vi "SortAndNormalise.vi"(0 "Resampler":T1, 1 "ResampleToN":i32=12, 2 "ResampleHeights":dbl[](array[numeric])=[25.4, 38.1, 50.8, 76.2, 101.6, 127.0, 152.4, 203.2, 254.0, 304.8, 406.4, 508.0, 609.6, 812.8, 1219.2, 1524.0], 5 "Plot Array In":cluster{"Array":dbl[], "Array":dbl[]}[](array[cluster]), 7 "LegendsIn":string[](array[string]), 9 "Use for:":T2(array[ring])=[enum."\nU", enum."\nLambda", enum."\nTI", enum."\nSigma"], 12 "Zref":dbl) -> (4 "SortedLegends":string[](array[string]), 6 "SortedData":cluster{"Array":dbl[], "Array":dbl[]}[](array[cluster]), 8 "LeftGraph":cluster{"Array":dbl[], "Array":dbl[]}[](array[cluster]), 10 "RightGraph":cluster{"Array":dbl[], "Array":dbl[]}[](array[cluster]), 14 "UzClusterOutput":cluster{"Array":dbl[], "Array":dbl[]})   [LabVIEW 2021]
uses:
  Resampler.ctl
panel:
  # "Fit using values at  measurement Z heights"
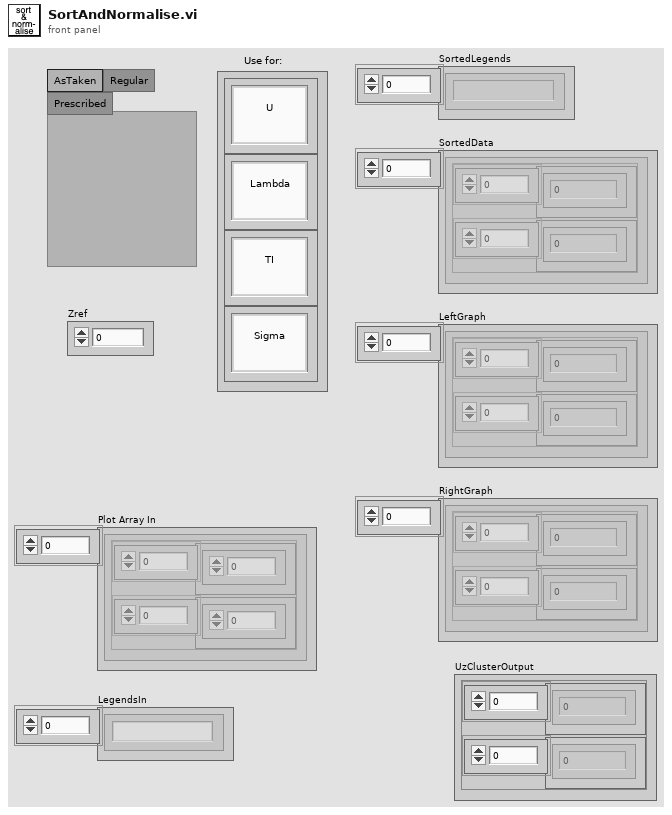
[diagram p1: front panel]
types:
  T1 = typedef "Resampler.ctl" = enum32{"AsTaken", "Regular", "Prescribed"}
  T2 = enum16{"Don't Use", "\nU", "\nLambda", "\nTI", "\nSigma"}[]
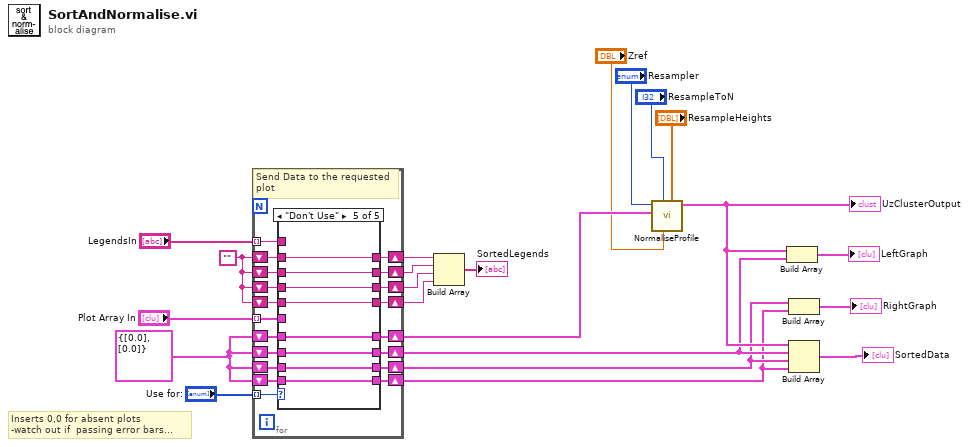
[diagram p0: block diagram]
diagram:
  w5 = cluster{dbl[], dbl[]} {[0.0], [0.0]}
  w11 = ""
  # "Inserts 0,0 for absent plots\n-watch out if  passing error bars..."
  n1 = for {
    tunnel: "Use for:" -> [w36] mode=indexing
    shift-right: [w41] -> w3
    shift-left: w5 -> [w35]
    shift-right: [w38] -> w2
    shift-left: w5 -> [w34]
    shift-right: [w37] -> w1
    shift-left: w5 -> [w33]
    shift-right: [w39] -> w18
    shift-left: w5 -> [w40]
    tunnel: "Plot Array In" -> [w32] mode=indexing
    tunnel: "LegendsIn" -> [w30] mode=indexing
    shift-right: [w31] -> w15
    shift-left: w11 -> [w29]
    shift-right: [w25] -> w14
    shift-left: w11 -> [w24]
    shift-right: [w26] -> w13
    shift-left: w11 -> [w27]
    shift-right: [w28] -> w12
    shift-left: w11 -> [w23]
    # "Send Data to the requested plot"
    n2 = case shown="\"Don't Use\"" w36 {
      tunnel: [w49 w55 w63 w72 w81] -> w41
      tunnel: w40 -> [_ w54 w64 w73 w80]
      tunnel: [w46 w54 w64 w73 w80] -> w39
      tunnel: [w48 w57 w65 w71 w79] -> w38
      tunnel: [w47 w56 w62 w70 w78] -> w37
      tunnel: w35 -> [w49 _ w63 w72 w81]
      tunnel: w34 -> [w48 w57 _ w71 w79]
      tunnel: w33 -> [w47 w56 w62 _ w78]
      tunnel: w32 -> [w46 w55 w65 w70 _]
      tunnel: [w43 w50 w58 w69 w74] -> w31
      tunnel: w30 -> [w45 w53 w61 w69 _]
      tunnel: w29 -> [w43 w50 w58 _ w74]
      tunnel: [w45 w52 w60 w68 w77] -> w28
      tunnel: [w44 w53 w59 w67 w76] -> w26
      tunnel: w27 -> [w44 _ w59 w67 w76]
      tunnel: [w42 w51 w61 w66 w75] -> w25
      tunnel: w24 -> [w42 w51 _ w66 w75]
      tunnel: w23 -> [_ w52 w60 w68 w77]
      frame "\nU", Default {
      }
      frame "\nLambda" {
      }
      frame "\nTI" {
      }
      frame "\nSigma" {
      }
      frame "Don't Use" {
      }
    }
  }
  n3 = Build Array(w12, w13, w14, w15) -> (→"SortedLegends":string[])
  n4 = call "NormaliseProfile.vi"("ResampleHeights"="ResampleHeights", "Zref"="Zref", "ResampleToN"="ResampleToN", "UzClusterIn"=w18, "Resampler"="Resampler") -> ("UzClusterOutput"=w22:cluster{dbl[], dbl[]})  [unwired: 5 in, 1 out]
  "UzClusterOutput" <- w22
  n5 = Build Array(w22, w3) -> (→"LeftGraph":cluster{dbl[], dbl[]}[])
  n6 = Build Array(w2, w1) -> (→"RightGraph":cluster{dbl[], dbl[]}[])
  n7 = Build Array(w22, w3, w2, w1) -> (→"SortedData":cluster{dbl[], dbl[]}[])
